vi "Update Task Status.vi"(8 "error in (no error)":errorcluster, 9 "Status":string, 10 "Task Name":string, 11 "InfoService in":refnum<class "NodeStatus.lvclass">) -> (0 "error out":errorcluster, 3 "InfoService out":refnum<class "NodeStatus.lvclass">)   [LabVIEW 2020, in "Vecto.lvlib" / "NodeStatus.lvclass"]
uses:
  NodeStatus.lvclass
  Task Status Data.ctl
  NodeStatus.lvclass/NodeStatus.ctl
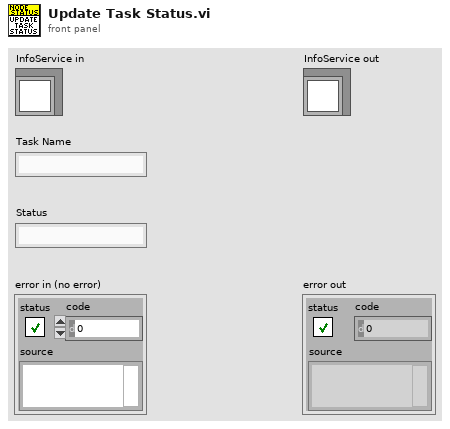
[diagram p1: front panel]
types:
  T1 = typedef "Vecto.lvlib/NodeStatus.lvclass/Task Status Data.ctl" = cluster{"Name":string, "Status":string}
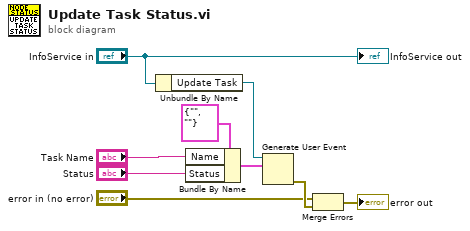
[diagram p0: block diagram]
diagram:
  n1 = Unbundle By Name("InfoService in") -> ("Update Task"=w9:refnum<user-event>)
  n2 = Bundle By Name(cluster=T1 {"Name"="", "Status"=""} ("event data"), "Name"="Task Name", "Status"="Status") -> (w7:T1)
  n3 = Generate User Event(user event=w9, event data cluster=w7) -> (error out=w4:errorcluster)  [unwired: 2 in, 1 out]
  n4 = Merge Errors("error in (no error)", w4) -> (→"error out":errorcluster)
  "InfoService out" <- "InfoService in"
